vi "Test_xmlread.vi"() -> ()   [LabVIEW 2013, in "VI-Test.lvlib"]
uses:
  lib/VI-Test.lvlib
  classes/Datastructure/Report/Report.lvclass
  lib/XML.lvlib
panel:
  out "Report (Ausgang)":refnum<class "Report.lvclass">
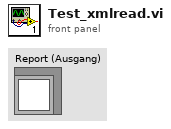
[diagram p1: front panel]
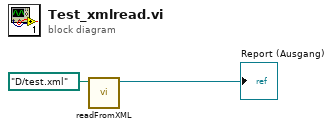
[diagram p0: block diagram]
diagram:
  n1 = call "readFromXML.vi"("file path (use dialog)"=path "D:/test.xml") -> ("Report (Ausgang)"=→"Report (Ausgang)":refnum<class "Report.lvclass">)  [unwired: 9 in, 1 out]
